vi "update_attrs.vi"(8 "error in (no error)":errorcluster, 10 "Nested Enqueuers Map":T1(c390), 11 "command_parser in":refnum<class "command_parser.lvclass">) -> (0 "error out":errorcluster, 3 "command_parser out":refnum<class "command_parser.lvclass">)   [LabVIEW 2025, in "command_parser.lvlib" / "command_parser.lvclass"]
uses:
  command_parser.lvclass
  <vilib>/ActorFramework/Message Enqueuer/Message Enqueuer.lvclass
  command_parser.lvclass/command_parser.ctl
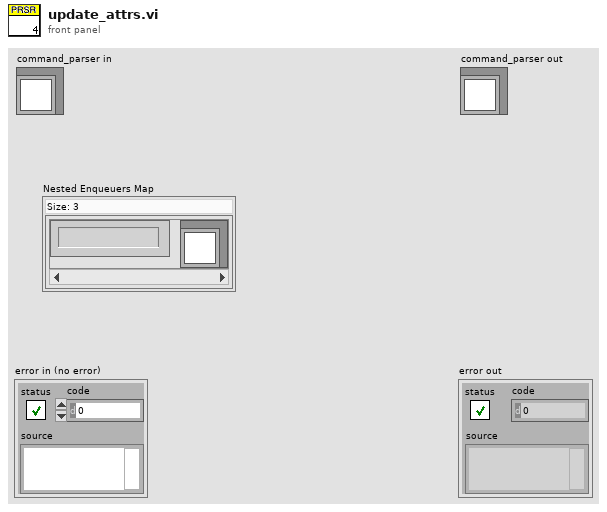
[diagram p1: front panel]
types:
  T1 = map{string, refnum<class "Message Enqueuer.lvclass">}
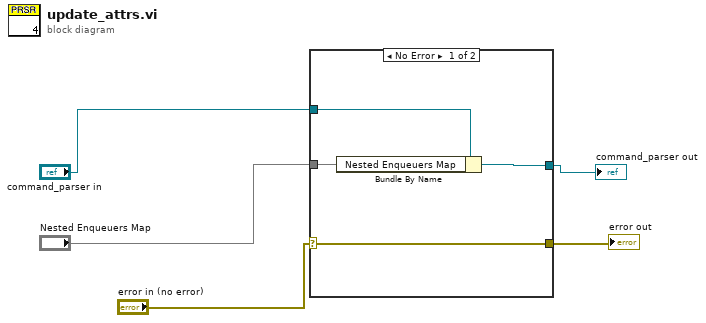
[diagram p0: block diagram]
diagram:
  n1 = case shown="No Error" "error in (no error)" {
    selector: "error in (no error)" -> [w6 w10]
    tunnel: "command_parser in" -> [w9 w11]
    tunnel: [w8 w11] -> w3
    tunnel: "Nested Enqueuers Map" -> [w7 _]
    tunnel: [w6 w10] -> w2
    frame No Error {
      n2 = Bundle By Name(cluster=w9, "Nested Enqueuers Map"=w7) -> (w8:refnum<class "command_parser.lvclass">)
    }
    frame Error {
    }
  }
  "error out" <- w2
  "command_parser out" <- w3
